vi "BB_SendAnglesDistanceTime.vi"(11 "Cluster":T1) -> ()   [LabVIEW 2012]
uses:
  typeDefs/targetVariables.ctl
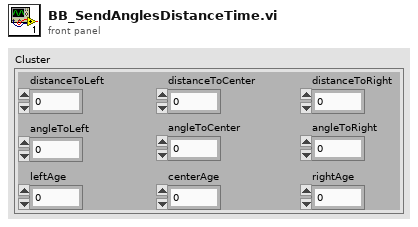
[diagram p1: front panel]
types:
  T1 = typedef "targetVariables.ctl" = cluster{"distanceToCenter":dbl, "angleToCenter":dbl, "angleToLeft":dbl, "distanceToLeft":dbl, "angleToRight":dbl, "distanceToRight":dbl, "centerAge":dbl, "leftAge":dbl, "rightAge":dbl}
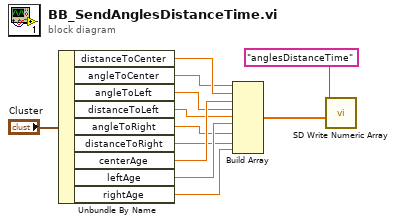
[diagram p0: block diagram]
diagram:
  n1 = Unbundle By Name("Cluster") -> ("distanceToCenter"=w6:dbl, "angleToCenter"=w5:dbl, "angleToLeft"=w4:dbl, "distanceToLeft"=w3:dbl, "angleToRight"=w2:dbl, "distanceToRight"=w1:dbl, "centerAge"=w10:dbl, "leftAge"=w9:dbl, "rightAge"=w8:dbl)
  n2 = Build Array(w5, w6, w10, w4, w3, w9, w2, w1, w8) -> (w11:dbl[])
  n3 = call <vilib>:"SD Write Numeric Array.vi"("Numeric Array"=w11, "Name"="anglesDistanceTime") -> ()  [unwired: 8 in, 2 out]
